vi "setup_lc_ly.vi"(0 "didian":string, 4 "shuoming":string, 6 "yongtu":string="领用", 7 "zc_luodi_num":string, 8 "yw":string, 10 "id":string) -> (2 "error":errorcluster caption="error out 2")   [LabVIEW 2017, in "Lib_code.lvlib"]
uses:
  Lib_code.lvlib
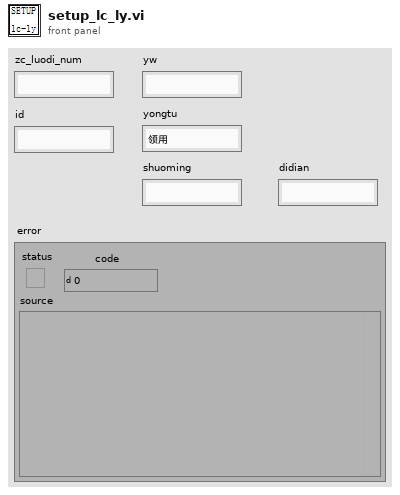
[diagram p1: front panel]
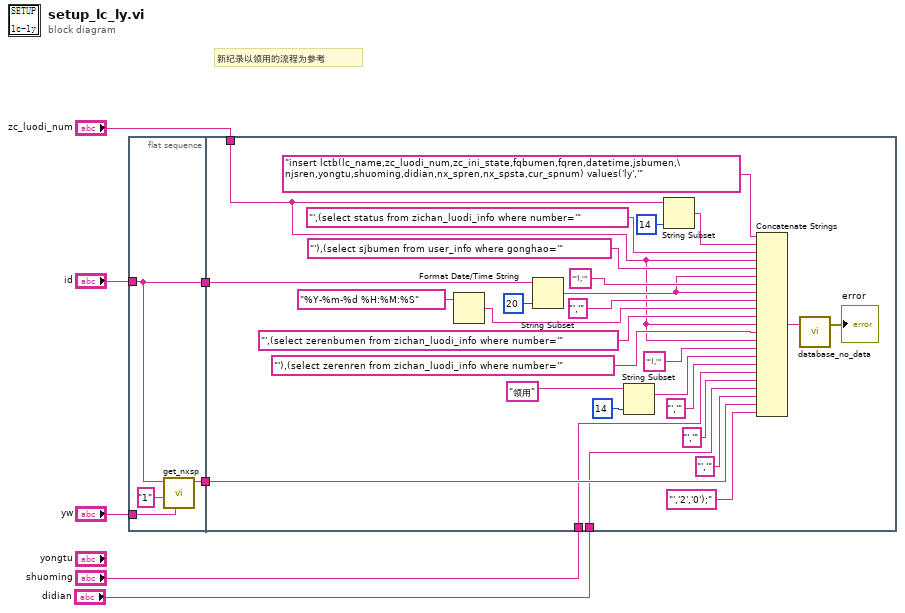
[diagram p0: block diagram]
diagram:
  # "新纪录以领用的流程为参考"
  n1 = flat-sequence {
    tunnel: "id" -> [w10]
    tunnel: [w10] -> w6
    tunnel: [w11] -> w5
    tunnel: "yw" -> [w9]
    tunnel: w6 -> [w17]
    tunnel: w5 -> [w28]
    tunnel: "zc_luodi_num" -> [w13]
    tunnel: "shuoming" -> [w25]
    tunnel: "didian" -> [w20]
    frame #0 {
      n2 = call "get_nxsp.vi"("yw"=w9, "Cur_state"="1", "fqren"=w10) -> ("sp_gonghao"=w11:string)  [unwired: 6 in, 2 out]
    }
    frame #1 {
      n3 = Format Date/Time String(time format string (%c)="%Y-%m-%d %H:%M:%S" ("时间格式字符串(%c)")) -> (date/time string=w18:string)  [unwired: 2 in]
      n4 = String Subset(string=w17, length (rest)=20 ("长度（剩余）")) -> (substring=w16:string)  [unwired: 1 in]
      n5 = String Subset(string="领用" ("字符串"), length (rest)=14 ("长度（剩余）")) -> (substring=w30:string)  [unwired: 1 in]
      n6 = String Subset(string=w13, length (rest)=14 ("长度（剩余）")) -> (substring=w37:string)  [unwired: 1 in]
      n7 = Concatenate Strings("insert lctb(lc_name,zc_luodi_num,zc_ini_state,fqbumen,fqren,datetime,jsbumen,\njsren,yongtu,shuoming,didian,nx_spren,nx_spsta,cur_spnum) values('ly','" ("格式字符串"), w37, "',(select status from zichan_luodi_info where number='" ("字符串"), w13, "'),(select sjbumen from user_info where gonghao='" ("字符串"), w16, "'),'" ("字符串"), w16, "','" ("字符串"), w18, "',(select zerenbumen from zichan_luodi_info where number='" ("字符串"), w13, "'),(select zerenren from zichan_luodi_info where number='" ("字符串"), w13, "'),'" ("字符串"), w30, "','" ("字符串"), w25, "','" ("字符串"), w20, "','" ("字符串"), w28, "','2','0');" ("字符串")) -> (w23:string)
      n8 = call "database_no_data.vi"("input"=w23) -> ("error"=→"error":errorcluster)  [unwired: 2 in]
    }
  }
